vi "Host_ExtendedDetails_Update.vi"(0 "reference in":refnum<vi>, 1 "Data array in":T1[](array[typedef]) {"Motor Data"."motorControllerState" items=["unknown"=1, "boot-up"=0, "stopped"=4, "operational"=5, "pre-operational"=127, "connection lost"=128]}, 3 "Enum":enum16{"cRIO/IMU", "BMS", "MotorController"}(ring)) -> ()   [LabVIEW 2018]
doc: "Updates Health Check Display inside ExtendedDetails.vi"
uses:
  Master/DAQ/Master_DataControl.ctl
  Master/DAQ/TypeDef_cRIOData.ctl
  Master/IMU/TypeDef_IMUData.ctl
  Master/CAN/TypeDef_BMSData.ctl
  Master/CAN/TypeDef_BMS_Status.ctl
  Master/CAN/MotorController/fixedMotorData.ctl
  Master/CAN/MotorController/Type_Def MotorStatus.ctl
  <vilib>/Utility/miscctls.llb/LVRowAndColumnTypeDef.ctl
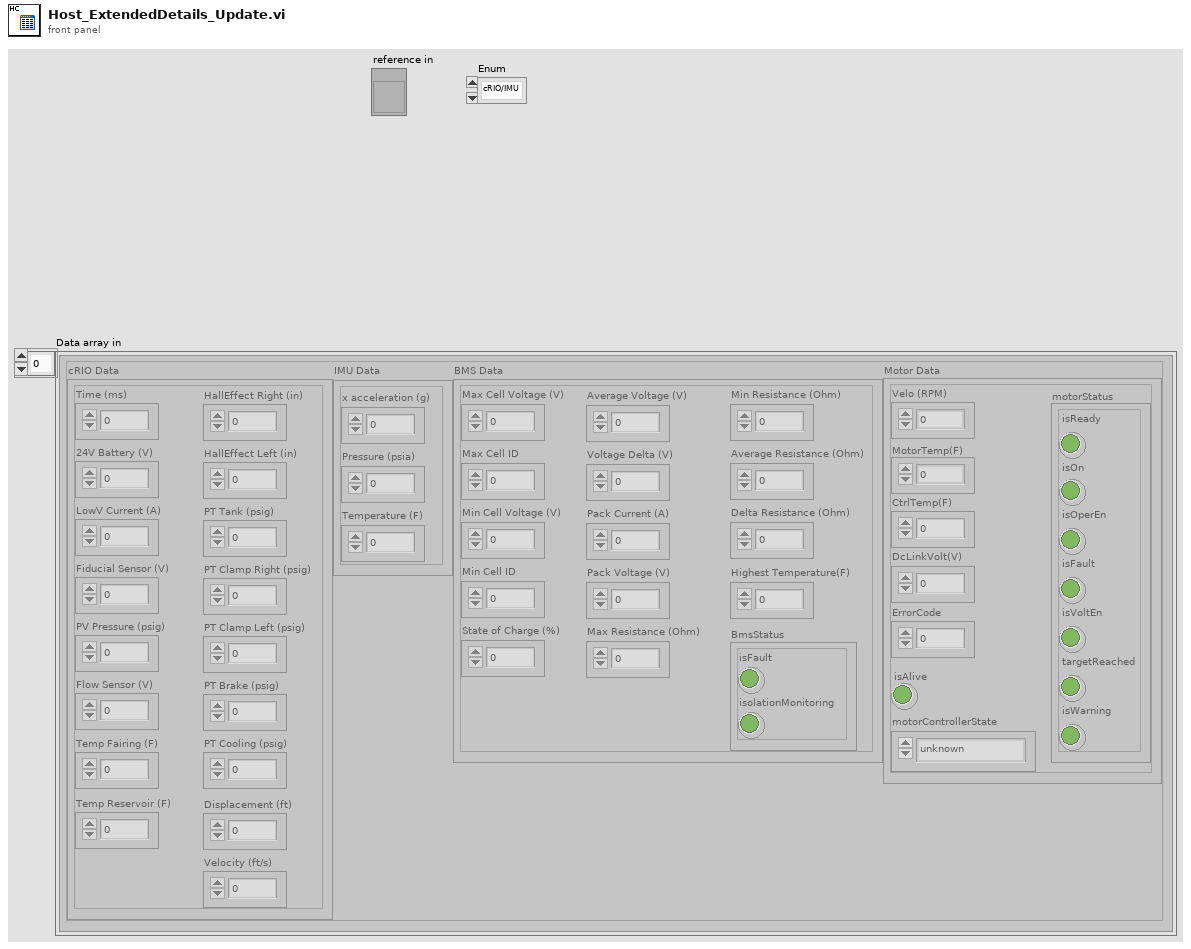
[diagram p1: front panel]
types:
  T1 = typedef "Master_DataControl.ctl" = cluster{"cRIO Data":T2, "IMU Data":T3, "BMS Data":T4, "Motor Data":T6}
  T2 = typedef "TypeDef_cRIOData.ctl" = cluster{"Time (ms)":dbl, "24V Battery (V)":dbl, "LowV Current (A)":dbl, "Fiducial Sensor (V)":dbl, "PV Pressure (psig)":dbl, "Flow Sensor (V)":dbl, "Temp Fairing (F)":dbl, "Temp Reservoir (F)":dbl, "HallEffect Right (in)":dbl, "HallEffect Left (in)":dbl, "PT Tank (psig)":dbl, "PT Clamp Right (psig)":dbl, "PT Clamp Left (psig)":dbl, "PT Brake (psig)":dbl, "PT Cooling (psig)":dbl, "Displacement (ft)":dbl, "Velocity (ft/s)":dbl}
  T3 = typedef "TypeDef_IMUData.ctl" = cluster{"x acceleration (g)":dbl, "Pressure (psia)":dbl, "Temperature (F)":dbl}
  T4 = typedef "TypeDef_BMSData.ctl" = cluster{"Max Cell Voltage (V)":dbl, "Max Cell ID":dbl, "Min Cell Voltage (V)":dbl, "Min Cell ID":dbl, "State of Charge (%)":dbl, "Average Voltage (V)":dbl, "Voltage Delta (V)":dbl, "Pack Current (A)":dbl, "Pack Voltage (V)":dbl, "Max Resistance (Ohm)":dbl, "Min Resistance (Ohm)":dbl, "Average Resistance (Ohm)":dbl, "Delta Resistance (Ohm)":dbl, "Highest Temperature(F)":dbl, "BmsStatus":T5}
  T5 = typedef "TypeDef_BMS_Status.ctl" = cluster{"isFault":bool, "isolationMonitoring":bool}
  T6 = typedef "fixedMotorData.ctl" = cluster{"Velo (RPM)":dbl, "MotorTemp(F)":dbl, "CtrlTemp(F)":dbl, "DcLinkVolt(V)":dbl, "ErrorCode":dbl, "motorStatus":T7, "isAlive":bool, "motorControllerState":u16}
  T7 = typedef "Type_Def MotorStatus.ctl" = cluster{"isReady":bool, "isOn":bool, "isOperEn":bool, "isFault":bool, "isVoltEn":bool, "targetReached":bool, "isWarning":bool}
  T8 = typedef "LVRowAndColumnTypeDef.ctl" = cluster{"Row":i32, "Column":i32}
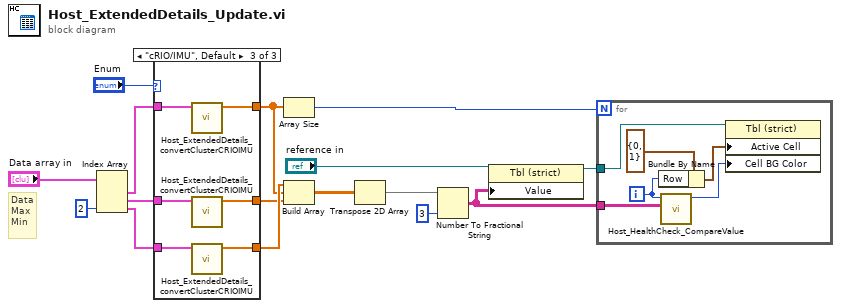
[diagram p0: block diagram]
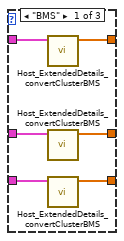
[diagram p2: hidden frame]
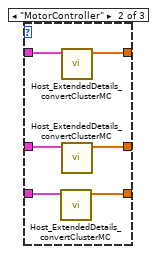
[diagram p3: hidden frame]
diagram:
  # "Data\nMax\nMin"
  n1 = Index Array(array="Data array in", index #3=2 ("index")) -> (element #1=w11:T1, element #2=w12:T1, element #3=w13:T1)  [unwired: 2 in]
  n2 = case shown="\"cRIO/IMU\", Default" "Enum" {
    tunnel: w13 -> [w17 w24 w34]
    tunnel: w12 -> [w20 w26 w33]
    tunnel: w11 -> [w22 w28 w32]
    tunnel: [w18 w23 w31] -> w10
    tunnel: [w19 w25 w30] -> w9
    tunnel: [w21 w27 w29] -> w8
    frame "BMS" {
      n3 = call "Host_ExtendedDetails_convertClusterBMS.vi"("Data"=w22) -> ("Array"=w21:dbl[])  [unwired: 10 in]
      n4 = call "Host_ExtendedDetails_convertClusterBMS.vi"("Data"=w20) -> ("Array"=w19:dbl[])  [unwired: 10 in]
      n5 = call "Host_ExtendedDetails_convertClusterBMS.vi"("Data"=w17) -> ("Array"=w18:dbl[])  [unwired: 10 in]
    }
    frame "MotorController" {
      n6 = call "Host_ExtendedDetails_convertClusterMC.vi"("Data"=w24) -> ("Array"=w23:dbl[])  [unwired: 10 in]
      n7 = call "Host_ExtendedDetails_convertClusterMC.vi"("Data"=w28) -> ("Array"=w27:dbl[])  [unwired: 10 in]
      n8 = call "Host_ExtendedDetails_convertClusterMC.vi"("Data"=w26) -> ("Array"=w25:dbl[])  [unwired: 10 in]
    }
    frame "cRIO/IMU", Default {
      n9 = call "Host_ExtendedDetails_convertClusterCRIOIMU.vi"("Data"=w32) -> ("appended array"=w29:dbl[])  [unwired: 10 in]
      n10 = call "Host_ExtendedDetails_convertClusterCRIOIMU.vi"("Data"=w33) -> ("appended array"=w30:dbl[])  [unwired: 10 in]
      n11 = call "Host_ExtendedDetails_convertClusterCRIOIMU.vi"("Data"=w34) -> ("appended array"=w31:dbl[])  [unwired: 10 in]
    }
  }
  n12 = Array Size(array=w8) -> (size(s)=w16:i32)
  n13 = Build Array(w10, w8, w9) -> (w4:dbl[][])
  n14 = Transpose 2D Array(2D array=w4) -> (transposed array=w3:dbl[][])
  n15 = Number To Fractional String(number=w3, precision (6)=i16 3) -> (F-format string=w7:string[][])  [unwired: 2 in]
  n16 = property on="Property Node" class="Tbl (strict)"(reference="reference in", "Value"=w7) -> (reference out=w15:refnum<vi>)  [unwired: 1 in, 1 out]
  n17 = for {
    N: w16 -> [_]
    tunnel: w15 -> [w36]
    tunnel: w7 -> [w35]
    i -> [w37]
    n18 = Bundle By Name(cluster=T8 {"Row"=0, "Column"=1} ("Active Cell:Active Cell"), "Row"=w37) -> (w39:T8)
    n19 = call "Host_HealthCheck_CompareValue.vi"("Table in"=w35, "Index"=w37) -> ("r/g"=w40:u32)  [unwired: 9 in]
    n20 = property on="Property Node" class="Tbl (strict)"(reference=w36, "Active Cell"=w39, "Cell BG Color"=w40) -> ()  [unwired: 1 in, 2 out]
  }
